vi "CS++Main.vi"() -> ()   [LabVIEW 2013]
doc: "This VI illustrates how to use the <b>Launch CS++StartActor.vi</b> as subVI.\n\nYou may create a copy and add your project specific stuff."
uses:
  Packages/CSPP_Core/Actors/CS++StartActor/CS++StartActor.lvlib
panel:
  out "Attributes found?":bool
  out "Error Out":errorcluster
  in  "Error In":errorcluster
  in  "CS++Factory":path
  in  "Start Actor":string
  in  "DB Connection String":string
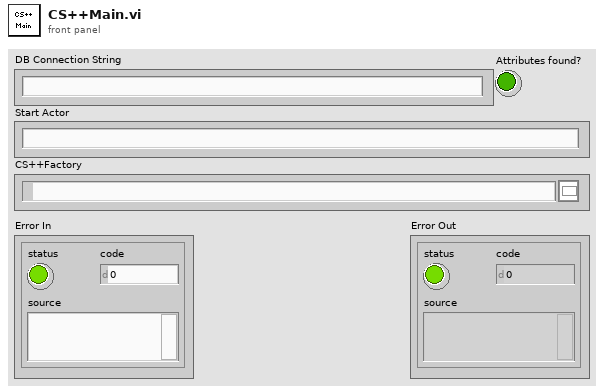
[diagram p1: front panel]
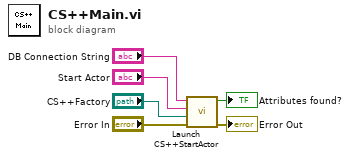
[diagram p0: block diagram]
diagram:
  n1 = call "Launch CS++StartActor.vi"("Error In"="Error In", "CS++Factory"="CS++Factory", "Start Actor"="Start Actor", "DB Connection String"="DB Connection String") -> ("Error Out"=→"Error Out":errorcluster, "Attributes found?"=→"Attributes found?":bool)  [unwired: 6 in]
